vi "Main.vi"() -> ()   [LabVIEW 2026]
doc: "The boiler controller allows a user to start and shut down a boiler.\nUse the Reset, Start, and Light Pilot controls to sequentially start the boiler.\nUse the Fuel Control Valve to change the flow of fuel into the boiler.\nUse the Stop Boiler button to shut down the boiler.\nTo shut down the system or in the event of an emergency, use the Emergency Stop button to close the application completely."
uses:
  controls/MHL Data.ctl
  controls/MHL UI Data.ctl
  controls/MHL Status.ctl
  controls/MHL References.ctl
  controls/MHL Configuration.ctl
  support/Boiler System Globals.vi
  support/Message Queue/Message Queue.lvlib
  support/User Event - Stop/User Event - Stop.lvlib
panel:
  out "Forced Draft Fan":bool
  out "Pilot":bool
  out "Pilot Gas Valve":bool
  out "Primary Fan":bool
  out "Status":string
  in  "Fuel Control Valve":u32(slide) scale=10.0..75.0
  in  "Emergency Stop":bool
  in  "Stop Boiler":bool
  in  "Light Pilot":bool
  in  "Start":bool
  in  "Reset":bool
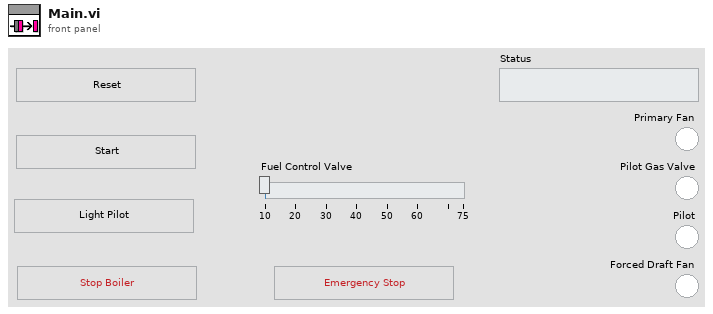
[diagram p1: front panel]
types:
  T1 = typedef "MHL Data.ctl" = cluster{"MHL User Interface Data":T2, "MHL References":T4, "MHL Configuration":T5}
  T2 = typedef "MHL UI Data.ctl" = cluster{"Status":string, "Fuel Control Valve":u32, "Primary Fan":bool, "Pilot Gas Valve":bool, "Pilot":bool, "Forced Draft Fan":bool, "MHL Status":T3}
  T3 = typedef "MHL Status.ctl" = enum16{"Lockout", "Ready", "Pre-Purge", "Pre-Purge Complete", "Pilot On", "Boiler Running", "Shutdown", "Purge"}
  T4 = typedef "MHL References.ctl" = cluster{"Reset Ref":refnum<vi>, "Start Ref":refnum<vi>, "Light Pilot Ref":refnum<vi>, "Stop Boiler Ref":refnum<vi>, "Fuel Control Valve Ref":refnum<vi>}
  T5 = typedef "MHL Configuration.ctl" = cluster{"Fuel Control Valve Maximum":dbl, "Fuel Control Valve Minimum":dbl}
  T6 = typedef "Notifiers.ctl" = cluster{"Handshake":refnum<notifier>, "Flame Level":refnum<notifier>, "Controller Exit":refnum<notifier>, "Boiler Ext":refnum<notifier>}
  T7 = typedef "Message Queue.lvlib/All Message Queues.ctl" = cluster{"MHL":refnum<queue>, "Boiler Controller":refnum<queue>}
  T8 = enum32{"invalid app kind", "Development System", "Run Time System", "Student Edition", "Embedded LabVIEW", "Evaluation", "Custom"}
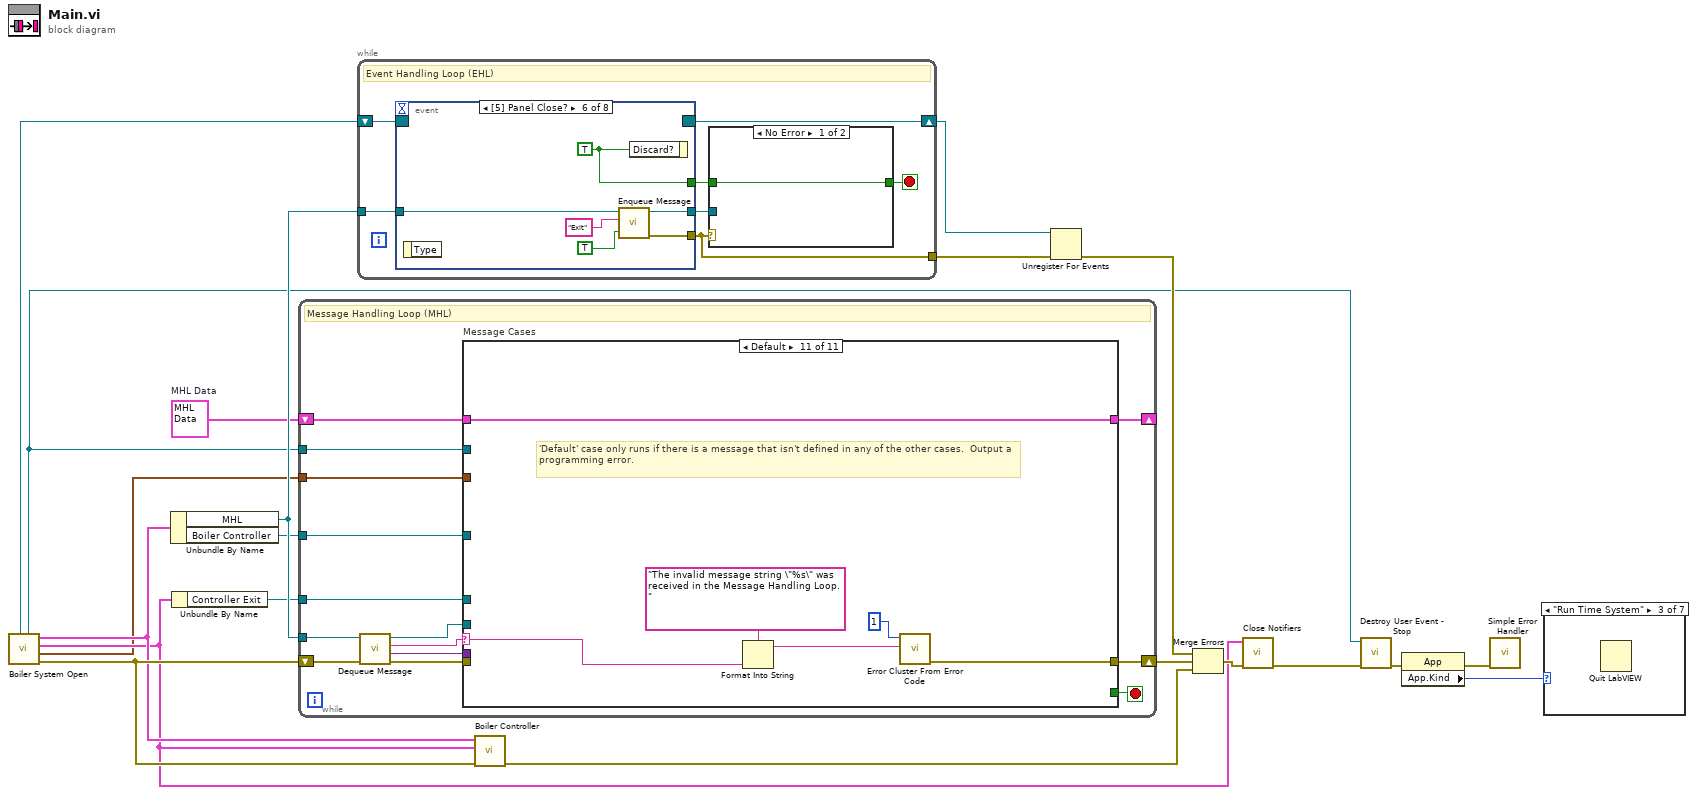
[diagram p0: block diagram]
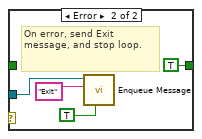
[diagram p8: hidden frame]
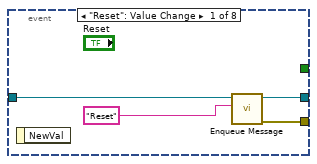
[diagram p9: hidden frame]
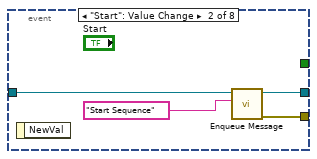
[diagram p10: hidden frame]
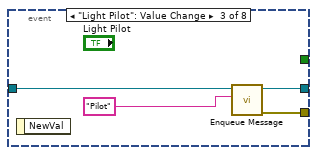
[diagram p11: hidden frame]
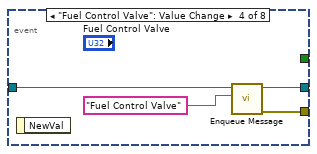
[diagram p12: hidden frame]
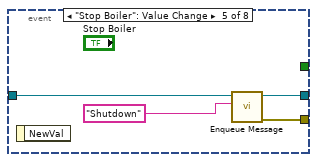
[diagram p13: hidden frame]
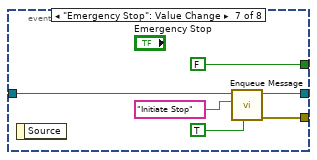
[diagram p14: hidden frame]
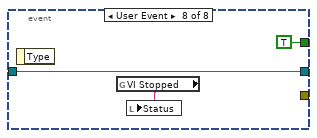
[diagram p15: hidden frame]
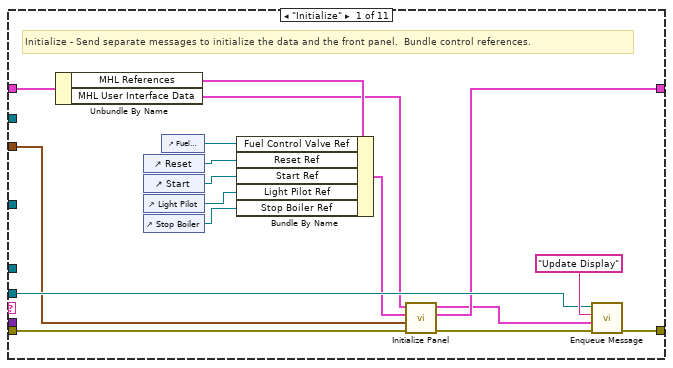
[diagram p16: hidden frame]
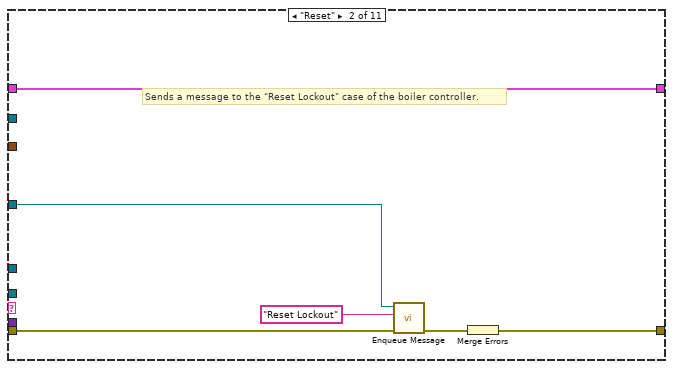
[diagram p17: hidden frame]
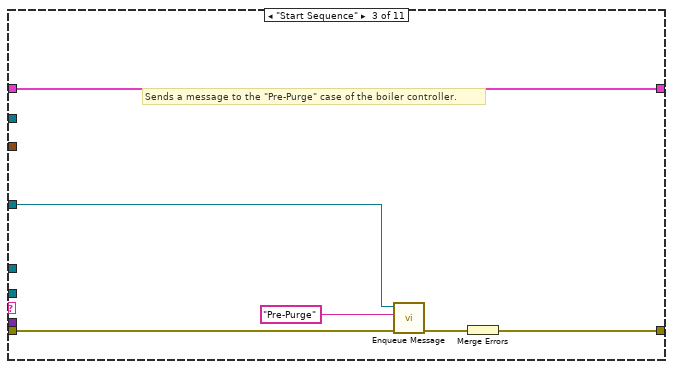
[diagram p18: hidden frame]
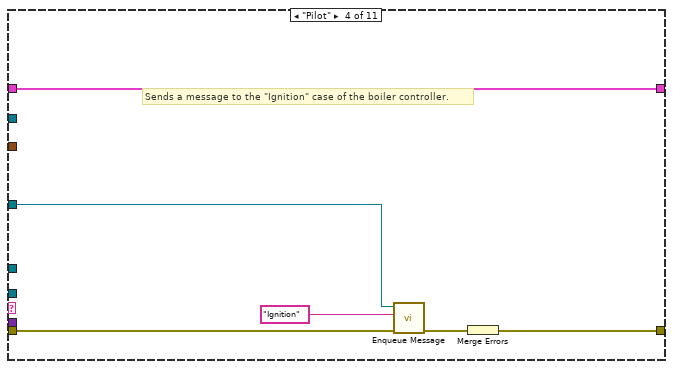
[diagram p19: hidden frame]
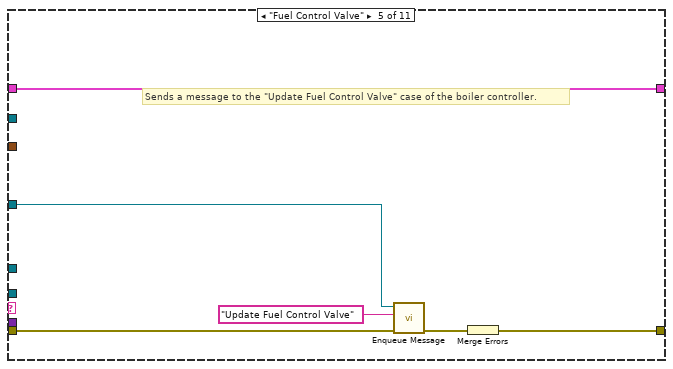
[diagram p20: hidden frame]
diagram:
  w2 = T1 {"MHL User Interface Data"={"Status"="", "Fuel Control Valve"=0, "Primary Fan"=FALSE, "Pilot Gas Valve"=FALSE, "Pilot"=FALSE, "Forced Draft Fan"=FALSE, "MHL Status"=enum."Lockout"}, "MHL References"={"Reset Ref"=refnum, "Start Ref"=refnum, "Light Pilot Ref"=refnum, "Stop Boiler Ref"=refnum, "Fuel Control Valve Ref"=refnum}, "MHL Configuration"={"Fuel Control Valve Maximum"=0.0, "Fuel Control Valve Minimum"=0.0}}  # MHL Data
  n1 = call "Boiler System Open.vi"() -> ("error out"=w8:errorcluster, "MHL Configuration"=w1:T5, "Notifiers"=w3:T6, "Message Queues"=w7:T7, "User Event - Stop"=w9:refnum<user-event>, "Stop Event Registration Refnum"=w10:refnum<event-registration>)  [unwired: 6 in]
  n2 = Unbundle By Name(w7) -> ("MHL"=w19:refnum<queue>, "Boiler Controller"=w15:refnum<queue>)
  n3 = Unbundle By Name(w3) -> ("Controller Exit"=w6:refnum<notifier>)
  n4 = while {
    tunnel: w19 -> [w24]
    shift-right: [w33] -> _
    shift-left: w2 -> [w34]
    tunnel: w9 -> [w30]
    shift-right: [w31] -> w20
    shift-left: w8 -> [w29]
    tunnel: w15 -> [w23]
    tunnel: w6 -> [w22]
    tunnel: w1 -> [w21]
    stop <- w32 stop-if-true
    # "Message Handling Loop (MHL)"
    n5 = call "Dequeue Message.vi"("error in"=w29, "Message Queue"=w24) -> ("error out"=w28:errorcluster, "Message Data"=w26:variant, "Message"=w27:string, "dup Message Queue"=w25:refnum<queue>)  [unwired: 6 in]
    n6 = case "Message Cases" shown="Default" w27 {
      selector: w27 -> [_ _ _ _ _ _ _ _ _ _ w131]
      tunnel: w25 -> [w42 _ _ _ _ _ _ w97 w113 w127 _]
      tunnel: w28 -> [w41 w55 w61 w67 w73 w79 w94 w102 w118 w122 _]
      tunnel: [w51 w56 w62 w68 w74 w80 w95 w96 w116 w123 w129] -> w31
      tunnel: w34 -> [w43 w57 w63 w69 w75 w81 w90 w103 w119 w126 w133]
      tunnel: [w36 w57 w63 w69 w75 w81 w83 w103 w119 w126 w133] -> w33
      tunnel: [_ _ _ _ _ _ _ _ _ TRUE _] -> w32
      tunnel: w26 -> [_ _ _ _ _ _ w93 _ _ _ _]
      tunnel: w30 -> [_ _ _ _ _ _ _ _ _ w121 _]
      tunnel: w23 -> [_ w52 w58 w64 w70 w76 _ _ w112 _ _]
      tunnel: w22 -> [_ _ _ _ _ _ _ w101 _ _ _]
      tunnel: w21 -> [w39 _ _ _ _ _ _ _ _ _ _]
      frame "Initialize" {
        # "Initialize - Send separate messages to initialize the data and the front panel.  Bundle control references."
        n7 = Unbundle By Name(w43) -> ("MHL References"=w49:T4, "MHL User Interface Data"=w37:T2)
        n8 = control-ref of="Reset"() -> (w47:refnum<vi>)
        n9 = control-ref of="Start"() -> (w46:refnum<vi>)
        n10 = control-ref of="Light Pilot"() -> (w45:refnum<vi>)
        n11 = control-ref of="Stop Boiler"() -> (w44:refnum<vi>)
        n12 = control-ref of="Fuel Control Valve"() -> (w48:refnum<vi>)
        n13 = Bundle By Name(cluster=w49, "Fuel Control Valve Ref"=w48, "Reset Ref"=w47, "Start Ref"=w46, "Light Pilot Ref"=w45, "Stop Boiler Ref"=w44) -> (w38:T4)
        n14 = call "Initialize Panel.vi"("error in"=w41, "MHL Configuration"=w39, "MHL References"=w38, "MHL UI Data in"=w37) -> ("error out"=w40:errorcluster, "MHL Data out"=w36:T1, "MHL UI Data out"=w35:T2)  [unwired: 5 in]
        n15 = call "Enqueue Message.vi"("error in"=w40, "Message Data"=w35, "Message"="Update Display", "Message Queue"=w42) -> ("error out"=w51:errorcluster)  [unwired: 6 in, 1 out]
      }
      frame "Reset" {
        # "Sends a message to the \"Reset Lockout\" case of the boiler controller."
        n16 = call "Enqueue Message.vi"("error in"=w55, "Message"="Reset Lockout", "Message Queue"=w52) -> ("error out"=w54:errorcluster)  [unwired: 7 in, 1 out]
        n17 = Merge Errors(w54) -> (w56:errorcluster)
      }
      frame "Start Sequence" {
        # "Sends a message to the \"Pre-Purge\" case of the boiler controller."
        n18 = call "Enqueue Message.vi"("error in"=w61, "Message"="Pre-Purge", "Message Queue"=w58) -> ("error out"=w60:errorcluster)  [unwired: 7 in, 1 out]
        n19 = Merge Errors(w60) -> (w62:errorcluster)
      }
      frame "Pilot" {
        # "Sends a message to the \"Ignition\" case of the boiler controller."
        n20 = call "Enqueue Message.vi"("error in"=w67, "Message"="Ignition", "Message Queue"=w64) -> ("error out"=w66:errorcluster)  [unwired: 7 in, 1 out]
        n21 = Merge Errors(w66) -> (w68:errorcluster)
      }
      frame "Fuel Control Valve" {
        # "Sends a message to the \"Update Fuel Control Valve\" case of the boiler controller."
        n22 = call "Enqueue Message.vi"("error in"=w73, "Message"="Update Fuel Control Valve", "Message Queue"=w70) -> ("error out"=w72:errorcluster)  [unwired: 7 in, 1 out]
        n23 = Merge Errors(w72) -> (w74:errorcluster)
      }
      frame "Shutdown" {
        # "Sends a message to the \"Shutdown\" case of the boiler controller."
        n24 = call "Enqueue Message.vi"("error in"=w79, "Message"="Shutdown", "Message Queue"=w76) -> ("error out"=w78:errorcluster)  [unwired: 7 in, 1 out]
        n25 = Merge Errors(w78) -> (w80:errorcluster)
      }
      frame "Update Display" {
        w91 = T2 {"Status"="", "Fuel Control Valve"=0, "Primary Fan"=FALSE, "Pilot Gas Valve"=FALSE, "Pilot"=FALSE, "Forced Draft Fan"=FALSE, "MHL Status"=enum."Lockout"}  # MHL UI Data
        # "Update Display - Convert the message data to a string to display in the Data Display indicator."
        n26 = Variant To Data(error in=w94, type=w91, Variant=w93) -> (data=w82:T2, error out=w92:errorcluster)
        n27 = Unbundle By Name(w82) -> ("Status"=→"Status":string, "Fuel Control Valve"=w88:u32, "Primary Fan"=→"Primary Fan":bool, "Pilot Gas Valve"=→"Pilot Gas Valve":bool, "Pilot"=→"Pilot":bool, "Forced Draft Fan"=→"Forced Draft Fan":bool)
        n28 = Bundle By Name(cluster=w90, "MHL User Interface Data"=w82) -> (w83:T1)
        n29 = local write "Fuel Control Valve"(w88) -> ()
        n30 = Merge Errors(w92) -> (w95:errorcluster)
      }
      frame "Wait on Boiler Exit" {
        n31 = Wait on Notification(notifier=w101, timeout in ms (-1)=10, error in (no error)=w102) -> (timed out?=w98:bool, error out=w99:errorcluster)  [unwired: 1 in, 2 out]
        n32 = case shown="False" w98 {
          tunnel: w99 -> [w106 w111]
          tunnel: w97 -> [w105 w110]
          tunnel: [w107 w109] -> w96
          frame False {
            n33 = call "Enqueue Message.vi"("error in"=w106, "Message"="Exit", "Message Queue"=w105) -> ("error out"=w107:errorcluster)  [unwired: 7 in, 1 out]
          }
          frame True {
            n34 = call "Enqueue Message.vi"("error in"=w111, "Message"="Wait on Boiler Exit", "Message Queue"=w110) -> ("error out"=w109:errorcluster)  [unwired: 7 in, 1 out]
          }
        }
      }
      frame "Initiate Stop" {
        # "When stopping, first send a message to stop the boiler controller.\nThen wait for the boiler and boiler controller to ext"
        n35 = call "Enqueue Message.vi"("error in"=w118, "Message"="Exit", "Message Queue"=w112) -> ("error out"=w117:errorcluster)  [unwired: 7 in, 1 out]
        n36 = call "Enqueue Message.vi"("error in"=w117, "Message"="Wait on Boiler Exit", "Message Queue"=w113) -> ("error out"=w116:errorcluster)  [unwired: 7 in, 1 out]
      }
      frame "Exit" {
        # "Stop the VI"
        # "Release the message queue reference"
        n37 = call "Fire User Event - Stop.vi"("User Event - Stop"=w121) -> ("error out"=w120:errorcluster)  [unwired: 10 in]
        n38 = Release Queue(queue=w127, error in (no error)=w122) -> (error out=w124:errorcluster)  [unwired: 1 in, 2 out]
        n39 = Merge Errors(w120, w124) -> (w123:errorcluster)
      }
      frame Default {
        # "'Default' case only runs if there is a message that isn't defined in any of the other cases.  Output a programming error."
        n40 = Format Into String(format string="The invalid message string \"%s\" was received in the Message Handling Loop." ("Unknown Message Error Text"), w131) -> (resulting string=w128:string)  [unwired: 2 in, 1 out]
        n41 = call <vilib>:"Error Cluster From Error Code.vi"("error message (\"\")"=w128, "error code (0)"=1) -> ("error out"=w129:errorcluster)  [unwired: 7 in]
      }
    }
  }
  n42 = while {
    tunnel: w19 -> [w140]
    tunnel: [w136] -> w17
    shift-right: [w134] -> w16
    shift-left: w10 -> [w135]
    stop <- w138 stop-if-true
    # "Event Handling Loop (EHL)"
    n43 = event shown="[5] Panel Close?" {
      selector: w135 -> [_ _ _ _ _ _ _ _]
      dyn-events: [_ _ _ _ _ _ _ _] -> w134
      timeout: _ -> [_ _ _ _ _ _ _ _]
      tunnel: [_ _ _ _ _ w171 FALSE ("Discard?") TRUE ("Discard?")] -> w139
      tunnel: w140 -> [w149 w153 w157 w161 w165 w170 w177 w180]
      tunnel: [w148 w152 w156 w160 w164 w169 w176 _] -> w136
      tunnel: [w147 w151 w155 w159 w163 w168 w174 w180] -> w137
      event "Reset": Value Change {
        n44 = event-data() -> ()  [unwired: 1 in, 1 out]
        n45 = call "Enqueue Message.vi"("Message"="Reset", "Message Queue"=w149) -> ("error out"=w148:errorcluster, "dup Message Queue"=w147:refnum<queue>)  [unwired: 8 in]
      }
      event "Start": Value Change {
        n46 = event-data() -> ()  [unwired: 1 in, 1 out]
        n47 = call "Enqueue Message.vi"("Message"="Start Sequence", "Message Queue"=w153) -> ("error out"=w152:errorcluster, "dup Message Queue"=w151:refnum<queue>)  [unwired: 8 in]
      }
      event "Light Pilot": Value Change {
        n48 = event-data() -> ()  [unwired: 1 in, 1 out]
        n49 = call "Enqueue Message.vi"("Message"="Pilot", "Message Queue"=w157) -> ("error out"=w156:errorcluster, "dup Message Queue"=w155:refnum<queue>)  [unwired: 8 in]
      }
      event "Fuel Control Valve": Value Change {
        n50 = event-data() -> ()  [unwired: 1 in, 1 out]
        n51 = call "Enqueue Message.vi"("Message"="Fuel Control Valve", "Message Queue"=w161) -> ("error out"=w160:errorcluster, "dup Message Queue"=w159:refnum<queue>)  [unwired: 8 in]
      }
      event "Stop Boiler": Value Change {
        n52 = event-data() -> ()  [unwired: 1 in, 1 out]
        n53 = call "Enqueue Message.vi"("Message"="Shutdown", "Message Queue"=w165) -> ("error out"=w164:errorcluster, "dup Message Queue"=w163:refnum<queue>)  [unwired: 8 in]
      }
      event Panel Close? {
        w171 = TRUE ("Discard?")
        n54 = event-data() -> ()  [unwired: 1 in, 1 out]
        n55 = call "Enqueue Message.vi"("Priority Message? (F)"=TRUE, "Message"="Exit", "Message Queue"=w170) -> ("error out"=w169:errorcluster, "dup Message Queue"=w168:refnum<queue>)  [unwired: 7 in]
        n56 = event-data("Discard?"=w171) -> ()  [unwired: 1 in, 1 out]
      }
      event "Emergency Stop": Value Change {
        n57 = event-data() -> ()  [unwired: 1 in, 1 out]
        n58 = call "Enqueue Message.vi"("Priority Message? (F)"=TRUE, "Message"="Initiate Stop", "Message Queue"=w177) -> ("error out"=w176:errorcluster, "dup Message Queue"=w174:refnum<queue>)  [unwired: 7 in]
      }
      event User Event {
        n59 = event-data() -> ()  [unwired: 1 in, 1 out]
        n60 = global read "Boiler System Globals.vi" "VI Stopped"() -> (w178:string)
        n61 = local write "Status"(w178) -> ()
      }
    }
    n62 = case shown="No Error" w136 {
      tunnel: [w141 TRUE ("Discard?")] -> w138
      tunnel: w139 -> [w141 _]
      tunnel: w137 -> [_ w144]
      frame No Error {
      }
      frame Error {
        # "On error, send Exit message, and stop loop."
        n63 = call "Enqueue Message.vi"("Priority Message? (F)"=TRUE, "Message"="Exit", "Message Queue"=w144) -> ()  [unwired: 7 in, 2 out]
      }
    }
  }
  n64 = call "Boiler Controller.vi"("error in"=w8, "Notifiers"=w3, "Message Queues"=w7) -> ("error out"=w14:errorcluster)  [unwired: 8 in]
  n65 = Unregister For Events(event registration refnum=w16, error in=w17) -> (error out=w18:errorcluster)
  n66 = Merge Errors(w18, w20, w14) -> (w5:errorcluster)
  n67 = call "Close Notifiers.vi"("error in"=w5, "Notifiers"=w3) -> ("error out"=w4:errorcluster)  [unwired: 9 in]
  n68 = call "Destroy User Event - Stop.vi"("error in"=w4, "User Event - Stop"=w9) -> ("error out"=w13:errorcluster)  [unwired: 9 in]
  n69 = property class="App"(error in=w13) -> (error out=w12:errorcluster, "App.Kind"=w11:T8)  [unwired: 1 in, 1 out]
  n70 = call <vilib>:"Simple Error Handler.vi"("error in (no error)"=w12) -> ()  [unwired: 4 in, 5 out]
  n71 = case shown="\"Run Time System\"" w11 {
    frame "invalid app kind", Default {
    }
    frame "Development System" {
    }
    frame "Run Time System" {
      n72 = Quit LabVIEW() -> ()  [unwired: 1 in]
    }
    frame "Student Edition" {
    }
    frame "Embedded LabVIEW" {
    }
    frame "Evaluation" {
    }
    frame "Custom" {
    }
  }
